vi "Split.vi"(6 "Groups":string[][](array[string]), 8 "error in (no error)":errorcluster caption="entrée d'erreur (pas d'erreur)", 9 "y":string[][](array[string]), 10 "X":string[][](array[string]), 11 "LeavePOut.lvclass":refnum<class "LeavePOut.lvclass">) -> (0 "error out":errorcluster caption="sortie d'erreur", 2 "Split":T1(array[cluster]), 3 "LeavePOut.lvclass":refnum<class "LeavePOut.lvclass">)   [LabVIEW 2020, in "LeavePOut.lvclass"]
doc: "Returns :\n \n- train : ndarray\n The training set indices for that split.\n\n- test : ndarray\n The testing set indices for that split."
uses:
  LeavePOut.lvclass
  LeavePOut.lvclass/LeavePOut.ctl
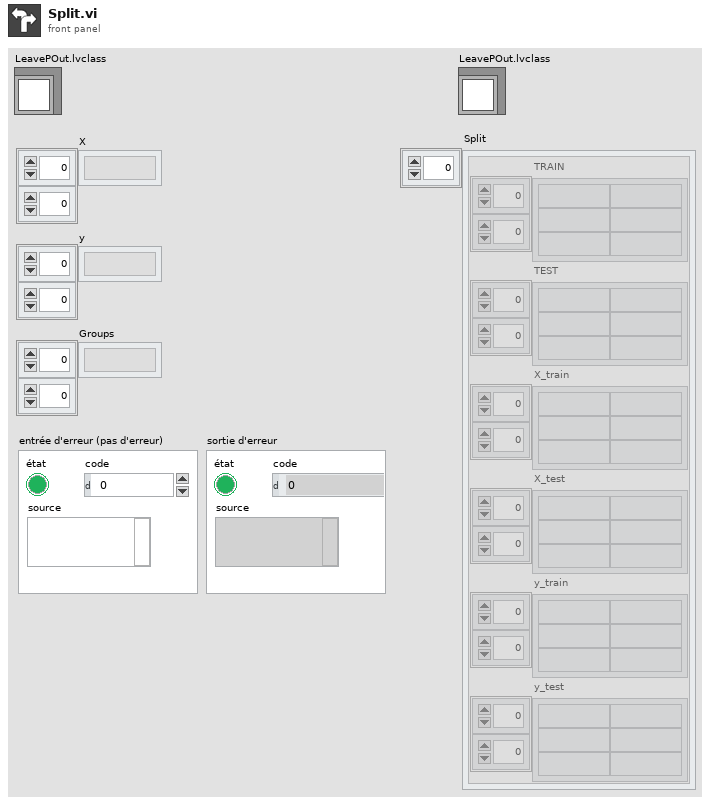
[diagram p1: front panel]
types:
  T1 = cluster{"TRAIN":string[][], "TEST":string[][], "X_train":string[][], "X_test":string[][], "y_train":string[][], "y_test":string[][]}[]
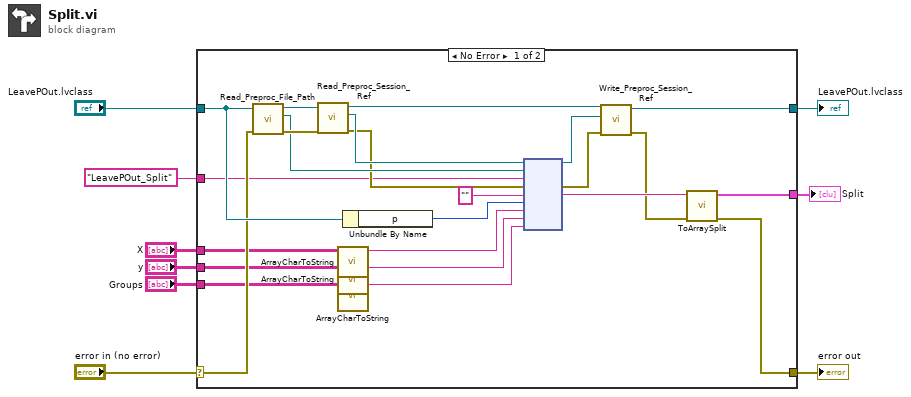
[diagram p0: block diagram]
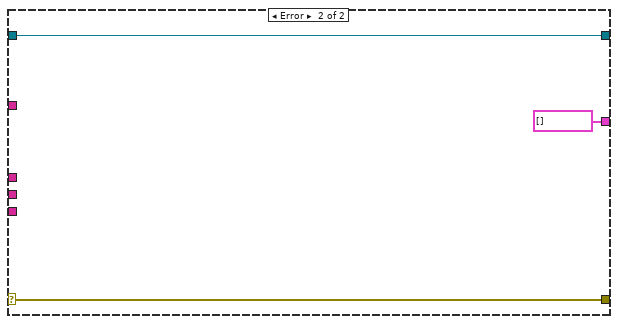
[diagram p2: hidden frame]
diagram:
  n1 = case shown="No Error" "error in (no error)" {
    selector: "error in (no error)" -> [w23 w36]
    tunnel: [w14 w36] -> w8
    tunnel: [w17 w35] -> w6
    tunnel: "LeavePOut.lvclass" -> [w24 w35]
    tunnel: "LeavePOut_Split" -> [w22 _]
    tunnel: "X" -> [w12 _]
    tunnel: "y" -> [w11 _]
    tunnel: "Groups" -> [w10 _]
    tunnel: [w13 T1 [] ("Split")] -> w1
    frame No Error {
      n2 = call-dynamic "Read_Preproc_File_Path.vi"("error in (no error)"=w23, "Python in"=w24) -> ("error out"=w32:errorcluster, "File_Path"=w31:path, "Python out"=w33:refnum<class "LeavePOut.lvclass">)  [unwired: 7 in]
      n3 = call-dynamic "Read_Preproc_Session_Ref.vi"("error in (no error)"=w32, "Python in"=w33) -> ("error out"=w29:errorcluster, "Session_ref"=w30:refnum<k35>, "Python out"=w28:refnum<class "LeavePOut.lvclass">)  [unwired: 7 in]
      n4 = call "ArrayCharToString.vi"("TAB"=w12) -> ("Instruction"=w20:string)  [unwired: 10 in]
      n5 = call "ArrayCharToString.vi"("TAB"=w11) -> ("Instruction"=w19:string)  [unwired: 10 in]
      n6 = call "ArrayCharToString.vi"("TAB"=w10) -> ("Instruction"=w18:string)  [unwired: 10 in]
      n7 = Unbundle By Name(w24) -> ("p"=w21:i32)
      n8 = node(w30, w31, w22, w29, "", w21, w20, w19, w18) -> (w26:refnum<k35>, w27:errorcluster, w16:string)  [unwired: 4 in, 2 out]
      n9 = call-dynamic "Write_Preproc_Session_Ref.vi"("error in (no error)"=w27, "Session_ref"=w26, "Python in"=w28) -> ("error out"=w15:errorcluster, "Python out"=w17:refnum<class "LeavePOut.lvclass">)  [unwired: 7 in]
      n10 = call "ToArraySplit.vi"("sortie d'erreur"=w15, "Return value"=w16) -> ("sortie d'erreur"=w14:errorcluster, "Split"=w13:T1)  [unwired: 8 in]
    }
    frame Error {
    }
  }
  "error out" <- w8
  "LeavePOut.lvclass" <- w6
  "Split" <- w1
